vi "Listbox Strings.vi"(8 "error in (no error)":errorcluster, 11 "Folder Item in":refnum<class "Folder Item.lvclass">) -> (0 "error out":errorcluster, 2 "ItemName":string, 3 "Folder Item out":refnum<class "Folder Item.lvclass">)   [LabVIEW 2020, in "BetterDragAndDropDemo.lvlib" / "Folder Item.lvclass"]
uses:
  Folder Item.lvclass
  Folder Item.lvclass/Folder Item.ctl
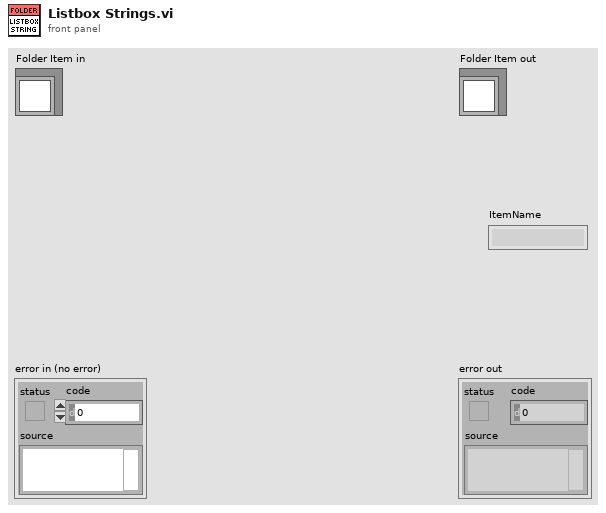
[diagram p1: front panel]
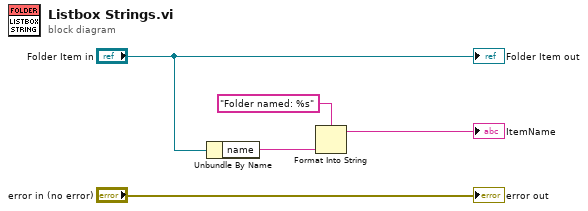
[diagram p0: block diagram]
diagram:
  n1 = Unbundle By Name("Folder Item in") -> ("name"=w3:string)
  n2 = Format Into String(format string="Folder named: %s", w3) -> (resulting string=→"ItemName":string)  [unwired: 2 in, 1 out]
  "error out" <- "error in (no error)"
  "Folder Item out" <- "Folder Item in"
